vi "Custom - RetainValues.vi"() -> ()   [LabVIEW 2012]
doc: "Sample numeric display item."
uses:
  <vilib>/NI Veristand/Display Template Support/Display Template Support.llb/cluster_Screen Item Settings.ctl
  <vilib>/NI Veristand/Display Template Support/Display Template Support.llb/cluster_Graph Scale Settings.ctl
  <vilib>/NI Veristand/Display Template Support/Display Template Support.llb/cluster_Graph Plot Settings.ctl
  <vilib>/NI Veristand/Display Template Support/Display Template Support.llb/enum_Display Template Handler Minimal To Widget Msg.ctl
  <vilib>/NI Veristand/Display Template Support/Display Template Support.llb/enum_Display Template Handler Minimal To Workspace.ctl
  <vilib>/NI Veristand/Display Template Support/Display Template Support.llb/sub_Display Template Handler Custom.vi
  <vilib>/NI Veristand/Execution/Workspace/NI VeriStand - Get Multiple Channel Values.vi
  <vilib>/NI Veristand/Execution/Workspace/NI_VS Workspace ExecutionAPI.lvlib
panel:
  out "Active System Definition File":path
  in  "Current Channels Monitored":i32(listbox)
  in  "Gateway IP Address":string
  in  "Item.Data":T1
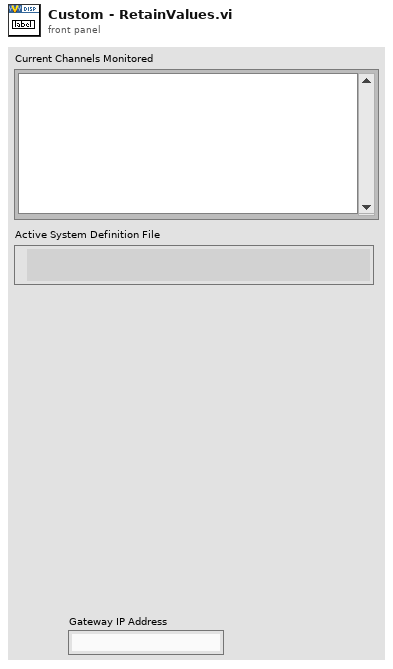
[diagram p1: front panel]
types:
  T1 = typedef "cluster_Screen Item Settings.ctl" = cluster{"Template VI":string, "Position X":i32, "Position Y":i32, "Custom":string, "Show Title Bar":bool, "ID":i32, "Always On Top":bool, "Allow Resize":bool, "Allow Minimize":bool, "Allow Close":bool, "Size to Screen":bool, "Screen.ID":i32, "State":enum16{"Normal", "New"}, "Title":string, "Window Bounds":cluster{"[0]":i16, "[1]":i16, "[2]":i16, "[3]":i16}, "Channel Ref":u64, "Unit":string, "Default Units?":bool, "Flash Limit?":bool, "Color 1":u32, "Color 2":u32, "Color 3":u32, "Color 4":u32, "Bck Color":u32, "Fore Color":u32, "Limit 1":dbl, "Limit 2":dbl, "Limit 3":dbl, "Limit 4":dbl, "Limit Mode 1":i32, "Limit Mode 2":i32, "Limit Mode 3":i32, "Limit Mode 4":i32, "Scale Precision":i32, "Scale Min":dbl, "Scale Max":dbl, "Format":i32, "Precision":i32, "Background Type":i32, "IDs":i32[], "Units":string[], "Labels":string[], "Scale Factor":dbl, "Scale Offset":dbl, "YScale Index":u32[], "XScale":T2, "YScales":T2[], "Plots":T3[], "Update Period":dbl, "History Length":dbl, "My.Ref":refnum<vi>, "Is Control?":bool, "Channel Paths":string[], "Custom Data":variant}
  T2 = typedef "cluster_Graph Scale Settings.ctl" = cluster{"Format":u8, "Precision":u8, "Fit":u8, "Label":string, "Use Default Label":bool, "Label Visible":bool, "Min":dbl, "Max":dbl}
  T3 = typedef "cluster_Graph Plot Settings.ctl" = cluster{"Bar Style":u8, "Fill To":i16, "Fill/PtColor":u32, "Line Style":u8, "Line Width":u8, "Color":u32, "Interp":u8, "Point Style":u8}
  T4 = typedef "enum_Display Template Handler Minimal To Workspace.ctl" = cluster{"Operation":enum16{"SetCustomData", "DeleteItem"}, "Data":variant}
  T5 = typedef "enum_Display Template Handler Minimal To Widget Msg.ctl" = enum16{"Stop", "LaunchConfigDialog"}
  T6 = cluster{"Channels":string[], "Path to System Definition File 2":path}
  T7 = typedef "NI_VS Workspace ExecutionAPI.lvlib/WorkspaceAPI.ctl" = refnum<k24>
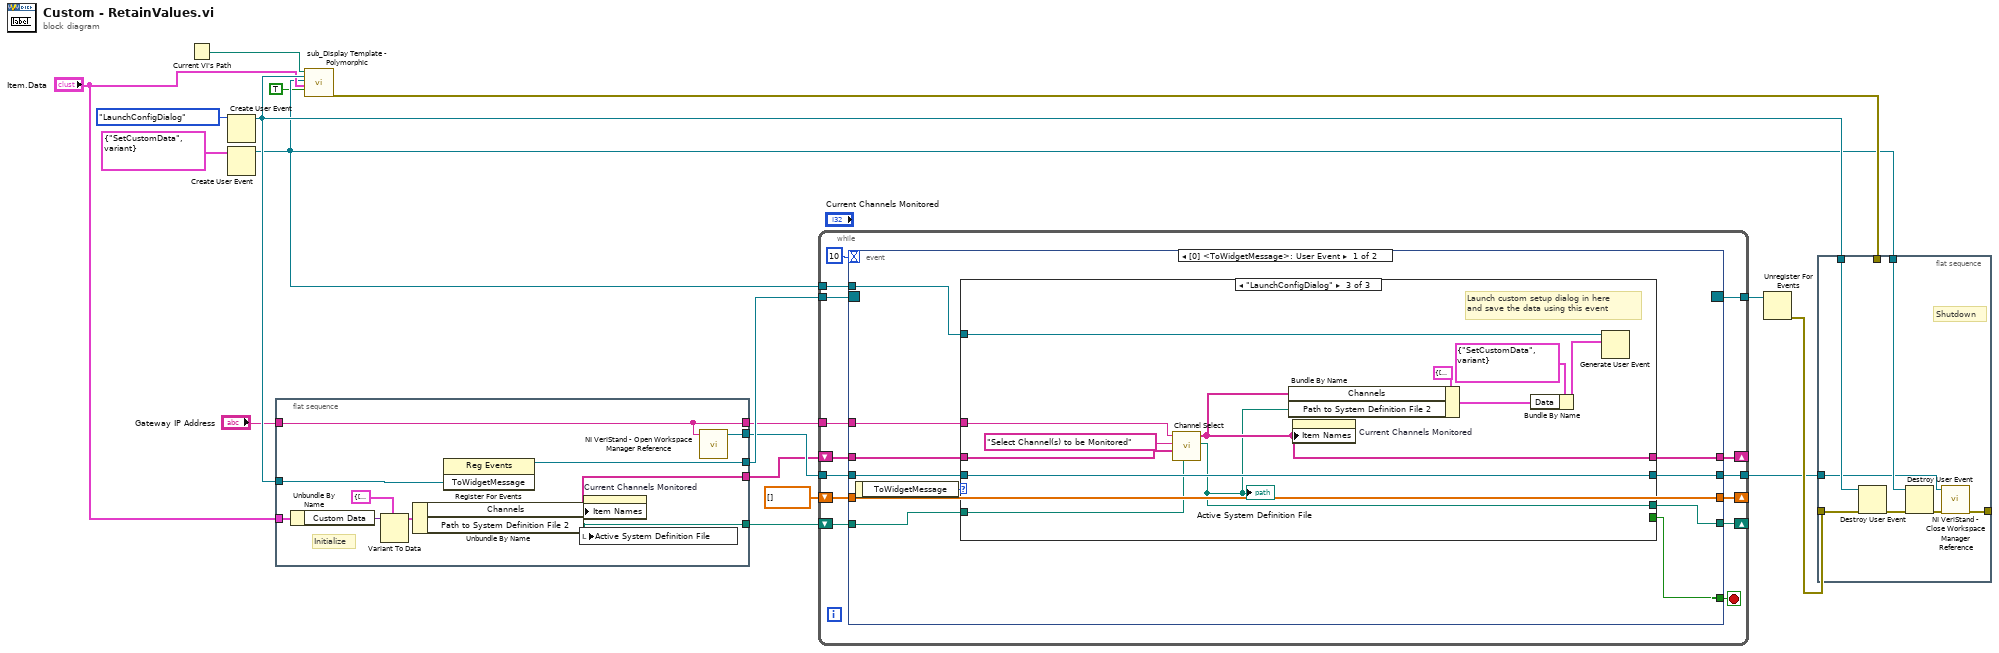
[diagram p0: block diagram]
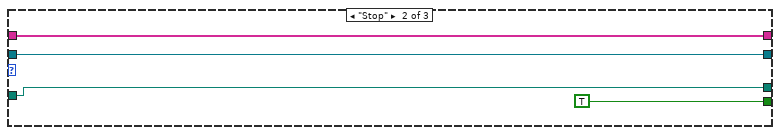
[diagram p3: hidden frame]
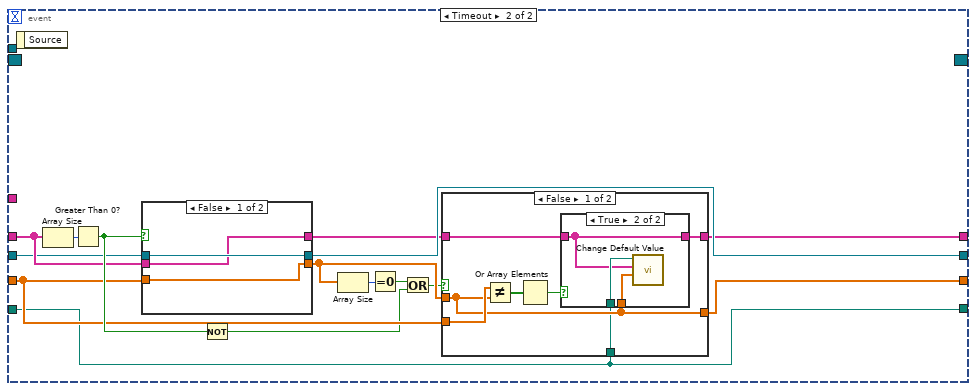
[diagram p4: hidden frame]
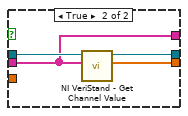
[diagram p7: hidden frame]
diagram:
  n1 = Current VI's Path() -> (path=w11:path)
  n2 = Create User Event(user event datatype=enum_Display_Template_Handler_Minimal_To_Widget_Msg."LaunchConfigDialog" ("ToWidgetMessage")) -> (user event=w13:refnum<user-event>)  [unwired: 1 in, 1 out]
  n3 = Create User Event(user event datatype=T4 {"Operation"=enum."SetCustomData", "Data"=variant} ("Data")) -> (user event=w9:refnum<user-event>)  [unwired: 1 in, 1 out]
  n4 = flat-sequence {
    tunnel: [w28] -> w16
    tunnel: w13 -> [w27]
    tunnel: "Item.Data" -> [w26]
    tunnel: "Gateway IP Address" -> [w24]
    tunnel: [w24] -> w6
    tunnel: [w23] -> w5
    tunnel: [w20] -> w2
    tunnel: [w19] -> w1
    frame #0 {
      # "Initialize"
      n5 = Unbundle By Name(w26) -> ("Custom Data"=w25:variant)
      n6 = Variant To Data(type=T6 {"Channels"=[], "Path to System Definition File 2"=path ""}, Variant=w25) -> (data=w21:T6)  [unwired: 1 in, 1 out]
      n7 = Unbundle By Name(w21) -> ("Channels"=w20:string[], "Path to System Definition File 2"=w19:path)
      n8 = register-events(w27) -> (reference out=w28:refnum<event-registration>)  [unwired: 2 in, 1 out]
      n9 = local write "Active System Definition File"(w19) -> ()
      n10 = property on="Current Channels Monitored" class="LstBox (strict)"("Item Names"=w20) -> ()  [unwired: 2 in, 2 out]
      n11 = call <vilib>:"NI VeriStand - Open Workspace Manager Reference.vi"("Gateway IP Address (\"\": localhost)"=w24) -> ("WorkspaceManager"=w23:T7)  [unwired: 9 in, 1 out]
    }
  }
  n12 = call-poly <vilib>:"sub_Display Template - Polymorphic.vi"("Parent.Path"=w11, "ToWidgetEvent"=w13, "ToWorkspace"=w9, "Item.Data"="Item.Data", "Resizable"=TRUE) -> ("error out"=w18:errorcluster)  [unwired: 1 in, 13 out]
  n13 = while {
    tunnel: w16 -> [w42]
    tunnel: [w40] -> w15
    tunnel: w9 -> [w39]
    tunnel: w6 -> [w38]
    tunnel: w5 -> [w36]
    tunnel: [w35] -> w3
    shift-right: [w34] -> _
    shift-left: w2 -> [w33]
    shift-right: [w32] -> _
    shift-left: dbl[] [] ("Values") -> [w31]
    shift-right: [w29] -> _
    shift-left: w1 -> [w30]
    stop <- w41 stop-if-true
    n14 = event shown="[0] <ToWidgetMessage>: User Event" {
      selector: w42 -> [_ _]
      dyn-events: [_ _] -> w40
      timeout: 10 -> [_ _]
      tunnel: [w52 _] -> w41
      tunnel: w39 -> [w51 _]
      tunnel: w38 -> [w50 _]
      tunnel: w36 -> [w49 w83]
      tunnel: [w48 w86] -> w35
      tunnel: [w47 w80] -> w34
      tunnel: w33 -> [w46 w84]
      tunnel: [w45 w81] -> w32
      tunnel: w31 -> [w45 w82]
      tunnel: w30 -> [w44 w79]
      tunnel: [w43 w79] -> w29
      event User Event {
        n15 = event-data() -> ("ToWidgetMessage"=w53:T5)  [unwired: 1 out]
        n16 = case shown="\"LaunchConfigDialog\"" w53 {
          tunnel: [_ TRUE _] -> w52
          tunnel: w51 -> [_ _ w72]
          tunnel: w50 -> [_ _ w71]
          tunnel: w49 -> [w56 w59 w67]
          tunnel: [w56 w59 w67] -> w48
          tunnel: [w55 w58 w63] -> w47
          tunnel: w46 -> [w55 w58 w66]
          tunnel: w44 -> [w54 w57 w65]
          tunnel: [w54 w57 w61] -> w43
          frame Default {
          }
          frame "Stop" {
          }
          frame "LaunchConfigDialog" {
            # "Launch custom setup dialog in here\nand save the data using this event"
            n17 = call "Channel Select.vi"("Path In"=w65, "Previous Selection"=w66, "Messaage"="Select Channel(s) to be Monitored", "Gateway IP Address"=w71) -> ("Path to System Definition File"=w61:path, "Channel Paths"=w63:string[])  [unwired: 5 in, 1 out]
            "Active System Definition File" <- w61
            n18 = Bundle By Name(cluster=T6 {"Channels"=[], "Path to System Definition File 2"=path ""}, "Channels"=w63, "Path to System Definition File 2"=w61) -> (w62:T6)
            n19 = property on="Current Channels Monitored" class="LstBox (strict)"("Item Names"=w63) -> ()  [unwired: 2 in, 2 out]
            n20 = Bundle By Name(cluster=T4 {"Operation"=enum."SetCustomData", "Data"=variant} ("event data"), "Data"=w62) -> (w68:T4)
            n21 = Generate User Event(user event=w72, event data cluster=w68) -> ()  [unwired: 1 in, 2 out]
          }
        }
      }
      event Timeout {
        n22 = event-data() -> ()  [unwired: 2 out]
        n23 = Array Size(array=w84) -> (size(s)=w87:i32)
        n24 = Greater Than 0?(x=w87) -> (x > 0?=w85:bool)
        n25 = case shown="False" w85 {
          tunnel: w83 -> [w103 w107]
          tunnel: w84 -> [w101 w104]
          tunnel: [w103 w106] -> w86
          tunnel: [w102 w105] -> w77
          tunnel: w82 -> [w102 _]
          tunnel: [w101 w104] -> w76
          frame False {
          }
          frame True {
            n26 = call-poly <vilib>:"NI VeriStand - Get Channel Value.vi"("Channels"=w104, "WorkspaceManager in"=w107) -> ("Values"=w105:dbl[], "WorkspaceManager out"=w106:T7)  [unwired: 7 in, 1 out]
          }
        }
        n27 = Not(x=w85) -> (.not. x?=w73:bool)
        n28 = Array Size(array=w77) -> (size(s)=w78:i32)
        n29 = Equal To 0?(x=w78) -> (x = 0?=w75:bool)
        n30 = Or(x=w75, y=w73) -> (x .or. y?=w74:bool)
        n31 = case shown="False" w74 {
          tunnel: w77 -> [w91 _]
          tunnel: w82 -> [w94 w100]
          tunnel: [w91 w100] -> w81
          tunnel: w76 -> [w92 w99]
          tunnel: [w88 w99] -> w80
          tunnel: w79 -> [w89 _]
          frame False {
            n32 = Not Equal?(x=w94, y=w91) -> (x != y?=w93:bool[])
            n33 = Or Array Elements(Boolean array=w93) -> (logical OR=w90:bool)
            n34 = case shown="True" w90 {
              tunnel: w92 -> [w95 w96]
              tunnel: w91 -> [_ w98]
              tunnel: w89 -> [_ w97]
              tunnel: [w95 w96] -> w88
              frame False {
              }
              frame True {
                n35 = call "Change Default Value.vi"("New Default Values"=w98, "Channels"=w96, "System Definition Path"=w97) -> ()  [unwired: 8 in, 1 out]
              }
            }
          }
          frame True {
          }
        }
      }
    }
  }
  n36 = Unregister For Events(event registration refnum=w15) -> (error out=w14:errorcluster)  [unwired: 1 in]
  n37 = flat-sequence {
    tunnel: w18 -> [_]
    tunnel: w14 -> [w113]
    tunnel: w13 -> [w114]
    tunnel: w9 -> [w111]
    tunnel: w3 -> [w109]
    tunnel: [w108] -> _
    frame #0 {
      # "Shutdown"
      n38 = Destroy User Event(user event=w114, error in=w113) -> (error out=w112:errorcluster)
      n39 = Destroy User Event(user event=w111, error in=w112) -> (error out=w110:errorcluster)
      n40 = call <vilib>:"NI VeriStand - Close Workspace Manager Reference.vi"("error in (no error)"=w110, "WorkspaceManager"=w109) -> ("error out"=w108:errorcluster)  [unwired: 9 in]
    }
  }
